vi "Get Dependencies.vi"(11 "VI Refnum":refnum<vi>) -> (1 "Get Missing Dependencies Information":T1, 2 "Dependency Paths":path[](array[path]), 3 "Dependency Names":string[](array[string]))   [LabVIEW 2017]
uses:
  <vilib>/Utility/miscctls.llb/LVMissingDepInfoTypeDef.ctl
panel:
  out "error out":errorcluster
  in  "error in":errorcluster
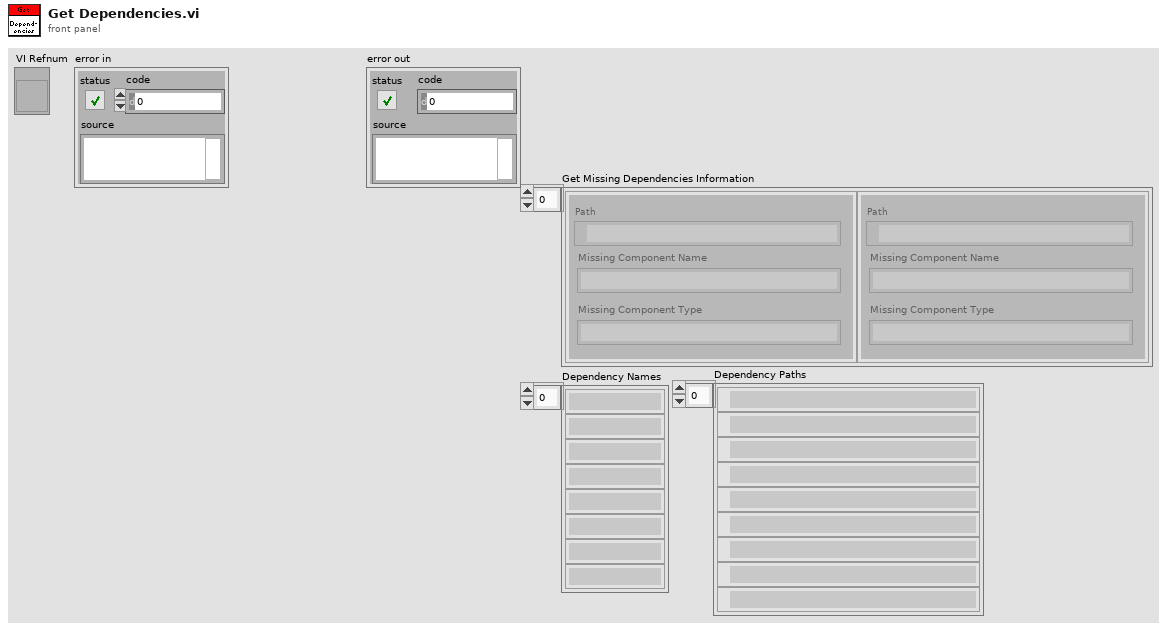
[diagram p1: front panel]
types:
  T1 = typedef "LVMissingDepInfoTypeDef.ctl" = cluster{"Path":path, "Missing Component Name":string, "Missing Component Type":string}[]
  T2 = enum8{"Only include commented out diagrams if diagram already loaded", "Never include commented out diagrams", "Always include commented out diagrams"}
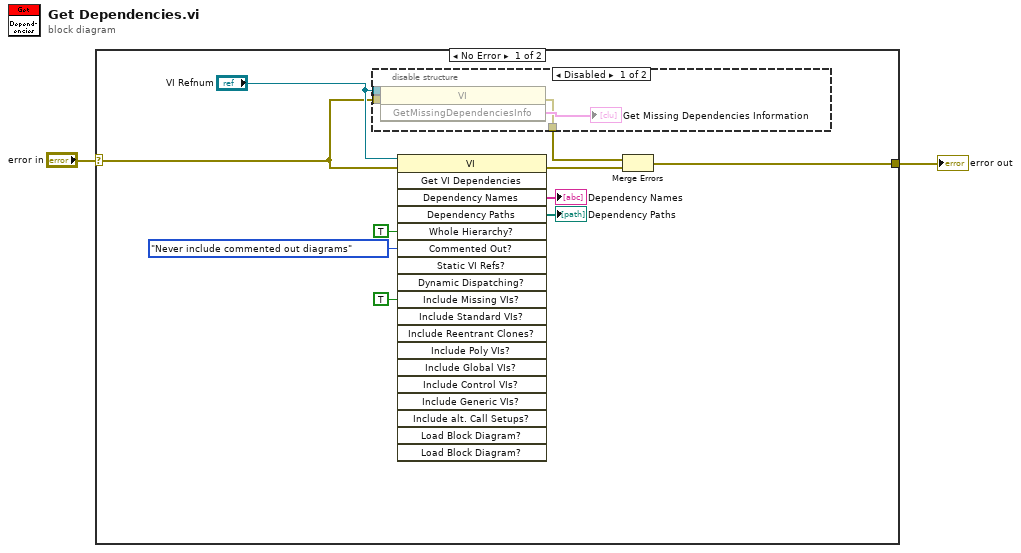
[diagram p0: block diagram]
diagram:
  n1 = case shown="No Error" "error in" {
    selector: "error in" -> [w3 w17]
    tunnel: [w5 w17] -> w2
    frame No Error {
      n2 = disable-structure shown="Disabled" {
        disable-tunnel: "VI Refnum" -> [w15 _]
        disable-tunnel: [w14 _] -> w4
        disable-tunnel: w3 -> [w13 _]
        frame Disabled {
          n3 = invoke class="VI" method="GetMissingDependenciesInfo"(reference=w15, error in=w13) -> (error out=w14:errorcluster, "GetMissingDependenciesInfo"=→"Get Missing Dependencies Information":T1)  [unwired: 1 in, 1 out]
        }
        frame Enabled {
        }
      }
      n4 = invoke class="VI" method="Get VI Dependencies"(reference="VI Refnum", error in=w3, "Whole Hierarchy?"=TRUE, "Commented Out?"=T2."Never include commented out diagrams" ("Commented Out Diagrams?"), "Include Missing VIs?"=TRUE ("Include Missing Items?")) -> (error out=w6:errorcluster, "Dependency Names"=→"Dependency Names":string[], "Dependency Paths"=→"Dependency Paths":path[])  [unwired: 14 in, 16 out]
      n5 = Merge Errors(w4, w6) -> (w5:errorcluster)
    }
    frame Error {
    }
  }
  "error out" <- w2
